vi "Arm_Down.vi"(10 "User Input":dbl, 11 "Numeric":dbl) -> ()   [LabVIEW 2012]
uses:
  Robot Global Data.vi
panel:
  in  "Arm Rate":dbl=-0.5
  # "Shoot"
  # "Down Hold time"
  # "Sec."
  # "Sec."
  # "UP / Down Time"
  # "+1/-1 Full Scale"
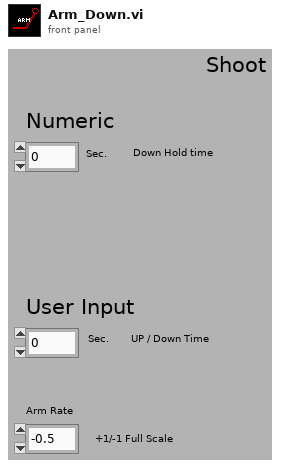
[diagram p1: front panel]
types:
  T1 = typedef "WPI_AnalogChannelDevRef.ctl" = cluster{"DevStatus":errorcluster, "Analog Module":T2, "Analog Channel":T3}
  T2 = typedef "FPGA_TypedefAnalogModule.ctl" = enum16{"Analog Module 1", "Analog Module 2"}
  T3 = typedef "FPGA_AIChannel.ctl" = enum8{"AI 1", "AI 2", "AI 3", "AI 4", "AI 5", "AI 6", "AI 7", "AI 8", "Invalid"}
  T4 = typedef "WPI_MotorControlDeviceRef.ctl" = cluster{"DeviceStatus":errorcluster, "Type":enum16{"PWM", "CAN"}, "PWM":cluster{"Digital Module":T5, "PWM Channel":T6, "DeadBand":T7}, "CAN":cluster{"Device Number":u8, "Control Mode":T8, "Semaphore":T9, "Max Vout":dbl}, "Invert":bool, "TransformRef":T10, "InvTransformRef":T10}
  T5 = typedef "FPGA_TypedefDigitalModule.ctl" = enum16{"Digital Module 1", "Digital Module 2"}
  T6 = typedef "FPGA_DIOPWMChannel.ctl" = enum8{"PWM 1", "PWM 2", "PWM 3", "PWM 4", "PWM 5", "PWM 6", "PWM 7", "PWM 8", "PWM 9", "PWM 10", "Invalid"}
  T7 = typedef "WPI_PWMDeadband.ctl" = cluster{"Name":string, "maxPositivePwm":i32, "minPositivePwm":i32, "centerPwm":i32, "maxNegativePwm":i32, "minNegativePwm":i32, "angularRange":u16}
  T8 = typedef "WPI_CANJaguar_ControlMode.ctl" = enum8{"Percent VBus", "Current", "Speed", "Position", "Voltage"}
  T9 = typedef "Semaphore RefNum" = refnum<k1>
  T10 = typedef "WPI_PWMTransform_ConPane.ctl" = refnum<vi>
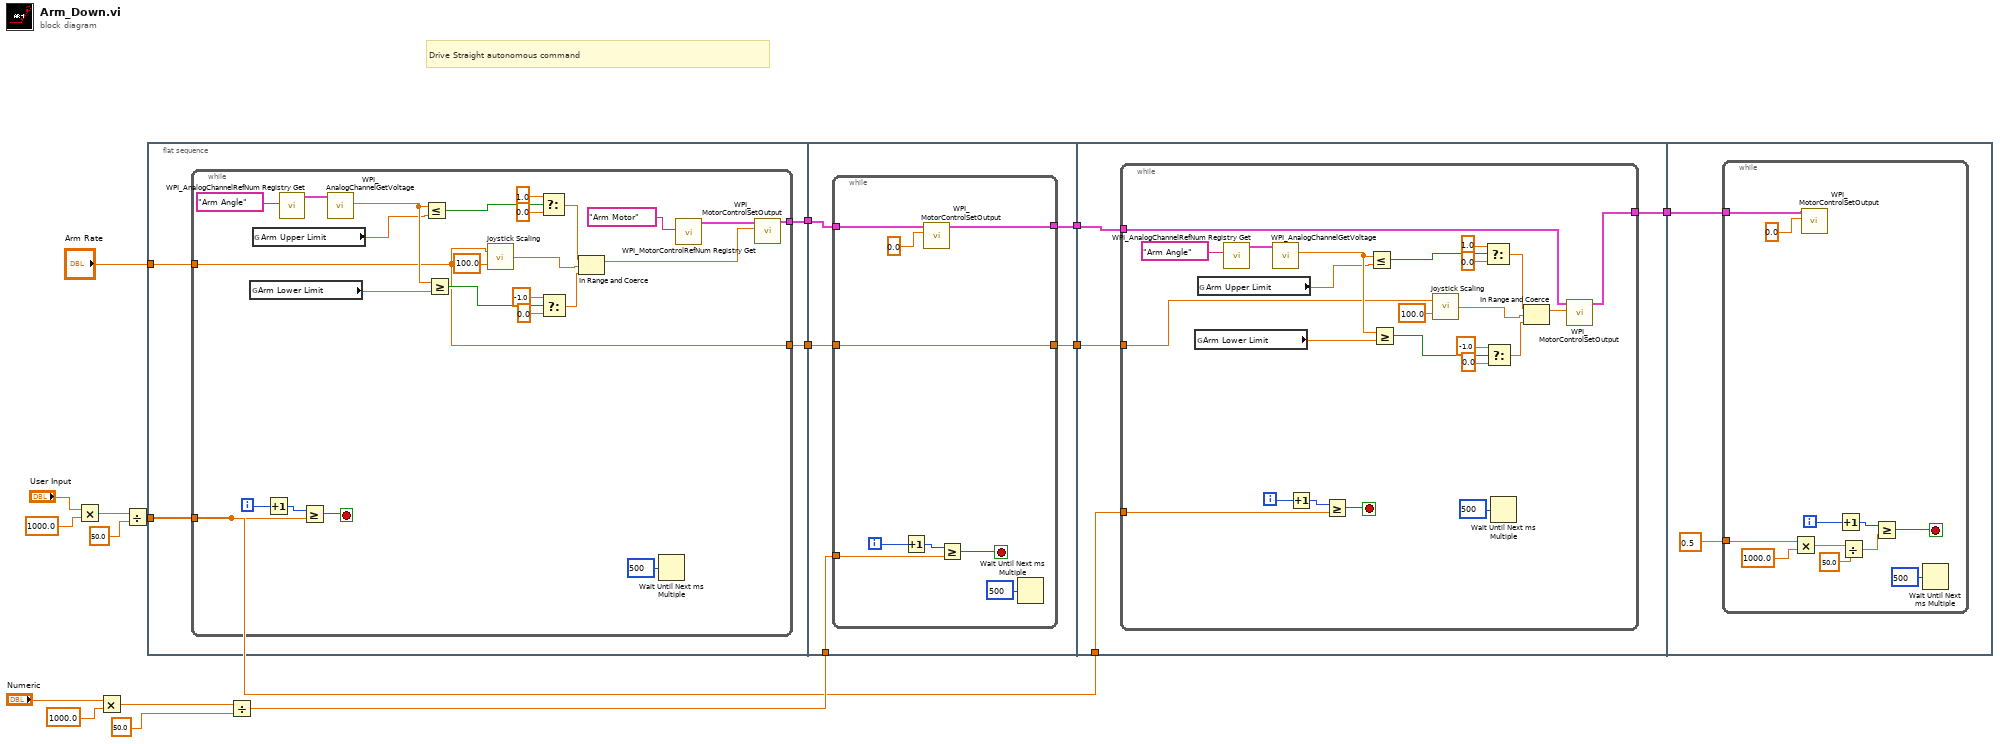
[diagram p0: block diagram]
diagram:
  # "Drive Straight autonomous command"
  n1 = Multiply(x="User Input", y=1000.0) -> (x*y=w15:dbl)
  n2 = Multiply(x="Numeric", y=1000.0) -> (x*y=w11:dbl)
  n3 = Divide(x=w15, y=50.0) -> (x/y=w5:dbl)
  n4 = flat-sequence {
    tunnel: w5 -> [w20]
    tunnel: [w19] -> w7
    tunnel: "Arm Rate" -> [w18]
    tunnel: [w17] -> w2
    tunnel: w8 -> [w50]
    tunnel: w7 -> [w49]
    tunnel: [w48] -> w6
    tunnel: w2 -> [w47]
    tunnel: [w46] -> w1
    tunnel: w6 -> [w63]
    tunnel: w5 -> [w62]
    tunnel: [w61] -> w4
    tunnel: w1 -> [w60]
    tunnel: w4 -> [w89]
    frame #0 {
      n5 = while {
        tunnel: w20 -> [w23]
        tunnel: [w22] -> w19
        tunnel: w18 -> [w21]
        tunnel: [w21] -> w17
        i -> [w24]
        stop <- w25 stop-if-true
        n6 = global read "Robot Global Data.vi" "Arm Lower Limit"() -> (w39:dbl)
        n7 = global read "Robot Global Data.vi" "Arm Upper Limit"() -> (w40:dbl)
        n8 = Increment(x=w24) -> (x+1=w26:i32)
        n9 = call <vilib>:"WPI_AnalogChannelRefNum Registry Get.vi"("refnum name"="Arm Angle") -> ("AIDeviceRef"=w42:T1)  [unwired: 9 in, 1 out]
        n10 = Greater Or Equal?(x=w26, y=w23) -> (x >= y?=w25:bool)
        n11 = call <vilib>:"WPI_AnalogChannelGetVoltage.vi"("AIDeviceRef"=w42) -> ("Voltage"=w41:dbl)  [unwired: 8 in, 2 out]
        n12 = Less Or Equal?(x=w41, y=w40) -> (x <= y?=w32:bool)
        n13 = Greater Or Equal?(x=w41, y=w39) -> (x >= y?=w31:bool)
        n14 = call "Joystick Scaling.vi"("Scale (%)"=100.0, "Input (+/- 1.00 volt)"=w21) -> ("Output"=w29:dbl)  [unwired: 1 in]
        n15 = Select(t=1.0, s=w32, f=0.0) -> (s? t:f=w37:dbl)
        n16 = Select(t=-1.0, s=w31, f=0.0) -> (s? t:f=w38:dbl)
        n17 = In Range and Coerce(upper limit=w37, x=w29, lower limit=w38) -> (coerced(x)=w30:dbl)  [unwired: 1 out]
        n18 = Wait Until Next ms Multiple(millisecond multiple=u32 500) -> ()  [unwired: 1 out]
        n19 = call <vilib>:"WPI_MotorControlRefNum Registry Get.vi"("refnum name"="Arm Motor") -> ("MotorControlDevRef"=w44:T4)  [unwired: 9 in, 1 out]
        n20 = call <vilib>:"WPI_MotorControlSetOutput.vi"("Output"=w30, "MotorControlDevRef"=w44) -> ("MotorControlDevRef"=w22:T4)  [unwired: 7 in, 2 out]
      }
    }
    frame #1 {
      n21 = while {
        tunnel: w50 -> [w55]
        tunnel: w49 -> [w54]
        tunnel: [w52] -> w48
        tunnel: w47 -> [w51]
        tunnel: [w51] -> w46
        i -> [w56]
        stop <- w57 stop-if-true
        n22 = Increment(x=w56) -> (x+1=w58:i32)
        n23 = call <vilib>:"WPI_MotorControlSetOutput.vi"("Output"=0.0, "MotorControlDevRef"=w54) -> ("MotorControlDevRef"=w52:T4)  [unwired: 7 in, 2 out]
        n24 = Greater Or Equal?(x=w58, y=w55) -> (x >= y?=w57:bool)
        n25 = Wait Until Next ms Multiple(millisecond multiple=u32 500) -> ()  [unwired: 1 out]
      }
    }
    frame #2 {
      n26 = while {
        tunnel: w62 -> [w67]
        tunnel: [w66] -> w61
        tunnel: w63 -> [w65]
        tunnel: w60 -> [w64]
        i -> [w68]
        stop <- w69 stop-if-true
        n27 = global read "Robot Global Data.vi" "Arm Lower Limit"() -> (w83:dbl)
        n28 = global read "Robot Global Data.vi" "Arm Upper Limit"() -> (w84:dbl)
        n29 = call <vilib>:"WPI_AnalogChannelRefNum Registry Get.vi"("refnum name"="Arm Angle") -> ("AIDeviceRef"=w86:T1)  [unwired: 9 in, 1 out]
        n30 = call <vilib>:"WPI_AnalogChannelGetVoltage.vi"("AIDeviceRef"=w86) -> ("Voltage"=w85:dbl)  [unwired: 8 in, 2 out]
        n31 = Increment(x=w68) -> (x+1=w70:i32)
        n32 = Greater Or Equal?(x=w70, y=w67) -> (x >= y?=w69:bool)
        n33 = Less Or Equal?(x=w85, y=w84) -> (x <= y?=w76:bool)
        n34 = Greater Or Equal?(x=w85, y=w83) -> (x >= y?=w75:bool)
        n35 = call "Joystick Scaling.vi"("Scale (%)"=100.0, "Input (+/- 1.00 volt)"=w64) -> ("Output"=w73:dbl)  [unwired: 1 in]
        n36 = Select(t=1.0, s=w76, f=0.0) -> (s? t:f=w81:dbl)
        n37 = Select(t=-1.0, s=w75, f=0.0) -> (s? t:f=w82:dbl)
        n38 = Wait Until Next ms Multiple(millisecond multiple=u32 500) -> ()  [unwired: 1 out]
        n39 = In Range and Coerce(upper limit=w81, x=w73, lower limit=w82) -> (coerced(x)=w74:dbl)  [unwired: 1 out]
        n40 = call <vilib>:"WPI_MotorControlSetOutput.vi"("Output"=w74, "MotorControlDevRef"=w65) -> ("MotorControlDevRef"=w66:T4)  [unwired: 7 in, 2 out]
      }
    }
    frame #3 {
      n41 = while {
        tunnel: 0.5 -> [w90]
        tunnel: w89 -> [w96]
        i -> [w97]
        stop <- w98 stop-if-true
        n42 = Multiply(x=w90, y=1000.0) -> (x*y=w93:dbl)
        n43 = call <vilib>:"WPI_MotorControlSetOutput.vi"("Output"=0.0, "MotorControlDevRef"=w96) -> ()  [unwired: 7 in, 3 out]
        n44 = Increment(x=w97) -> (x+1=w99:i32)
        n45 = Divide(x=w93, y=50.0) -> (x/y=w91:dbl)
        n46 = Greater Or Equal?(x=w99, y=w91) -> (x >= y?=w98:bool)
        n47 = Wait Until Next ms Multiple(millisecond multiple=u32 500) -> ()  [unwired: 1 out]
      }
    }
  }
  n48 = Divide(x=w11, y=50.0) -> (x/y=w8:dbl)
